vi "Set IR Emitter Power.vi"(0 "Session Handle in":T2, 5 "Emitter Power":T1=2 items=["2W"=2, "3W"=3, "4W"=4, "5W"=5], 11 "error in (no error)":errorcluster) -> (4 "Session Handle out":T2, 6 "Success?":bool, 15 "error out":errorcluster)   [LabVIEW 2015, in "PAS.lvclass"]
uses:
  PAS.lvclass
  Typedefs/Session Handle.ctl
  Typedefs/Emitter Power.ctl
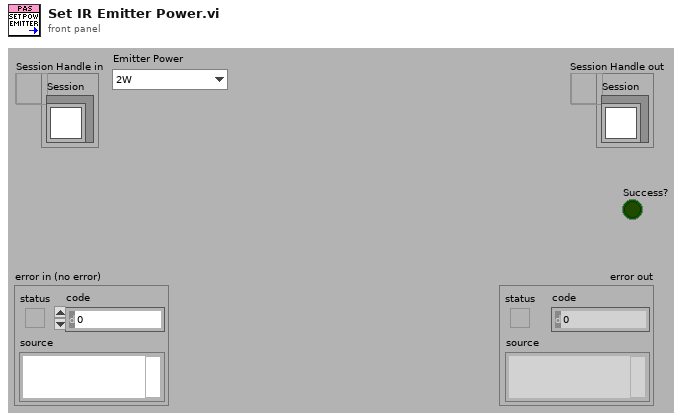
[diagram p1: front panel]
types:
  T1 = typedef "PAS.lvclass/Emitter Power.ctl" = u16
  T2 = typedef "PAS.lvclass/Session Handle.ctl" = refnum<data-value>
  T3 = typedef "XNET Frame CAN.ctl" = cluster{"timestamp":timestamp, "payload":u8[], "identifier":u32, "type":T4, "extended?":bool, "echo?":bool}
  T4 = typedef "XNET Frame Type CAN.ctl" = u8
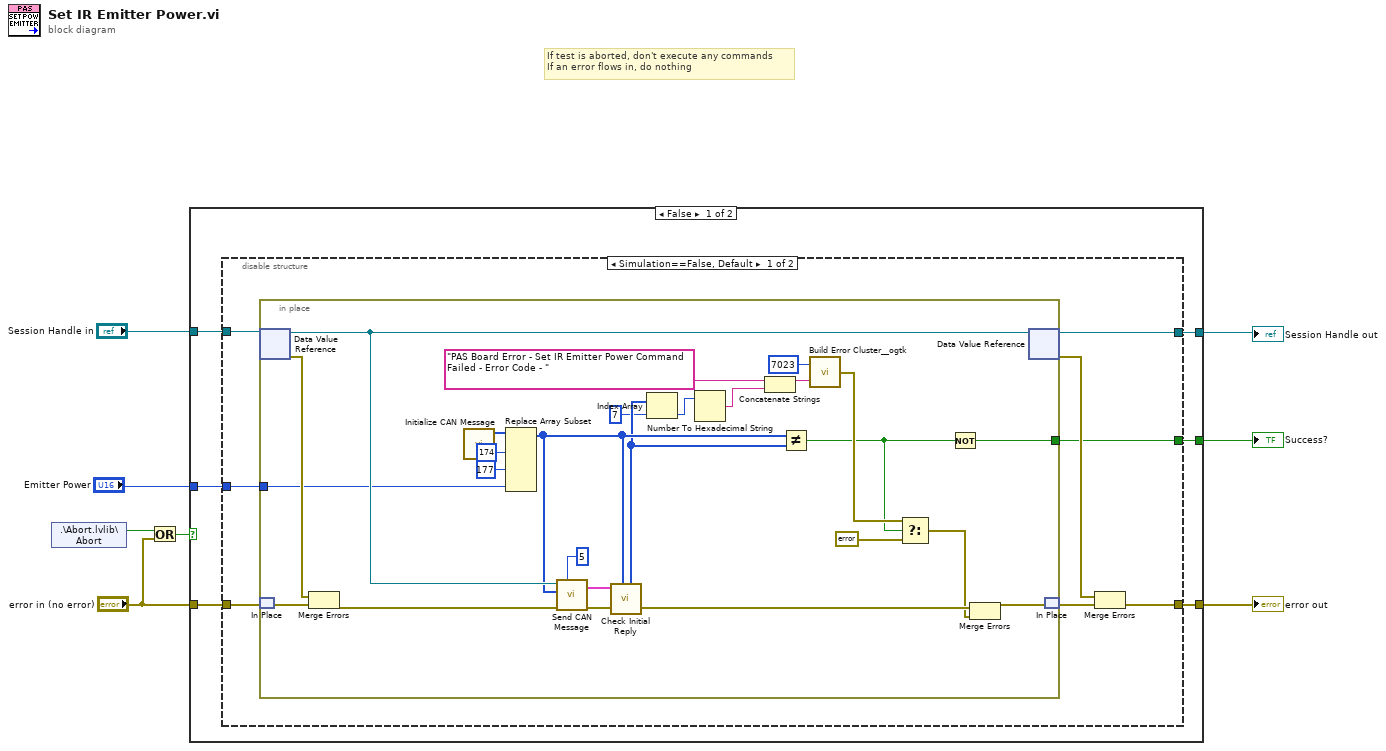
[diagram p0: block diagram]
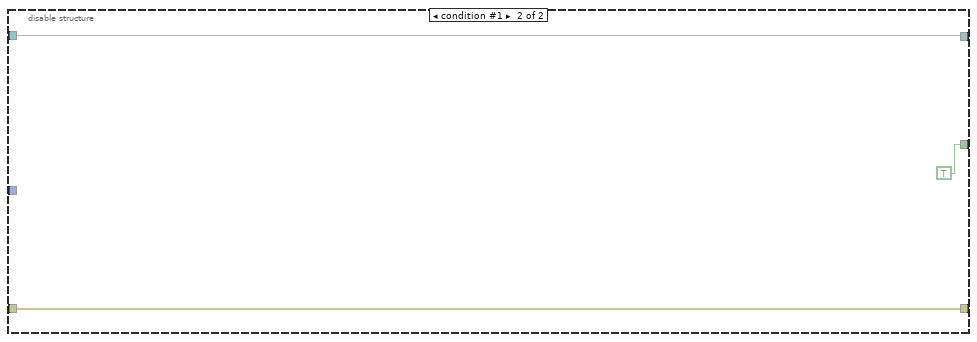
[diagram p2: hidden frame]
diagram:
  # "If test is aborted, don't execute any commands\nIf an error flows in, do nothing"
  n1 = shared-variable ".\\Abort.lvlib\\Abort"() -> (w5:bool)  [unwired: 1 in, 1 out]
  n2 = Or(x=w5, y="error in (no error)") -> (x .or. y?=w3:bool)
  n3 = case shown="False" w3 {
    tunnel: [w14 w52] -> w7
    tunnel: [w13 w51] -> w6
    tunnel: "Session Handle in" -> [w12 w52]
    tunnel: "error in (no error)" -> [w11 w51]
    tunnel: [w10 _] -> w2
    tunnel: "Emitter Power" -> [w9 _]
    frame False {
      n4 = disable-structure shown="Simulation==False, Default" {
        disable-tunnel: [w22 w50] -> w14
        disable-tunnel: [w19 w49] -> w13
        disable-tunnel: w12 -> [w18 w50]
        disable-tunnel: w11 -> [w17 w49]
        disable-tunnel: [w16 TRUE] -> w10
        disable-tunnel: w9 -> [w15 _]
        frame condition #0 (active) {
          n5 = in-place {
            in-place-border: [w34] -> w16
            in-place-border: w15 -> [w24]
            n6 = in-place-dvr #1(w18) -> (w41:refnum<class "PAS.lvclass">, w44:errorcluster)
            n7 = in-place-match #2(w17) -> (w43:errorcluster)
            n8 = Merge Errors(w44, w43) -> (w42:errorcluster)
            n9 = call "Initialize CAN Message.vi"() -> ("Initial Payload"=w45:u8[])  [unwired: 11 in]
            n10 = Replace Array Subset(array=w45, new element #1=u8 174 ("new element/subarray"), new element #2=u8 177 ("new element/subarray"), new element #3=w24) -> (w33:u8[])  [unwired: 3 in]
            n11 = call "Send CAN Message.vi"("Number of Retries"=5, "error in (no error)"=w42, "payload"=w33, "Gas In"=w41) -> ("error out"=w27:errorcluster, "Reply"=w39:T3[])  [unwired: 5 in, 1 out]
            n12 = call "Check Initial Reply.vi"("Write Message"=w33, "Reply"=w39) -> ("Whole Payload"=w32:u8[])  [unwired: 7 in, 2 out]
            n13 = Index Array(array=w32, index=7) -> (element=w30:u8)
            n14 = Number To Hexadecimal String(2:w30) -> (0:w29:string)  [unwired: 1 in]
            n15 = Concatenate Strings("PAS Board Error - Set IR Emitter Power Command Failed - Error Code - " ("string"), w29) -> (w28:string)
            n16 = Not Equal?(x=w33, y=w32) -> (x != y?=w35:bool)
            n17 = call <userlib>:"Build Error Cluster__ogtk.vi"("String to Prepend to source (\"\")"=w28, "code"=7023) -> ("error out"=w37:errorcluster)
            n18 = Select(t=w37, s=w35, f=errorcluster {"status"=FALSE, "code"=0, "source"=""}) -> (s? t:f=w26:errorcluster)
            n19 = Not(x=w35) -> (.not. x?=w34:bool)
            n20 = Merge Errors(w27, w26) -> (w46:errorcluster)
            n21 = in-place-dvr #1(w41) -> (w22:T2, w20:errorcluster)
            n22 = in-place-match #2(w46) -> (w21:errorcluster)
          }
          n23 = Merge Errors(w20, w21) -> (w19:errorcluster)
        }
        frame condition #1 {
        }
      }
    }
    frame True {
    }
  }
  "Session Handle out" <- w7
  "error out" <- w6
  "Success?" <- w2
